vi "Main interface manual control.vi"(1 "Current":T1={"Pump 1 control"={"Pump Direction"=0, "Flow rate (ml/min)"=1.0, "Target volum (ml)"=1.0, "Run"=FALSE}, "Pump 4 control"={"Pump Direction"=0, "Flow rate (ml/min)"=1.0, "Target volum (ml)"=1.0, "Run"=FALSE}, "Pump 2 control"={"Flowrate (ml/min)"=0.0, "Target volume (ml)"=0.0, "Run"=FALSE}, "Pump 5 control"={"Pump Direction"=0, "Flow rate (ml/min)"=1.0, "Target volum (ml)"=1.0, "Run"=FALSE}, "Pump 3 control"={"Flowrate (ml/min)"=0.0, "Target volume (ml)"=0.0, "Run"=FALSE}} {"Pump 3 control"."Target volume (ml)" min=0.0 max=50.0 format="%#.3g"; "Pump 3 control"."Flowrate (ml/min)" min=0.0 max=500.0 format="%#.3g"; "Pump 5 control"."Target volum (ml)" format="%#.4f"; "Pump 5 control"."Flow rate (ml/min)" format="%#.4f"; "Pump 5 control"."Pump Direction" items=["Infuse", "Withdraw"]; "Pump 2 control"."Target volume (ml)" min=0.0 max=50.0 format="%#.3g"; "Pump 2 control"."Flowrate (ml/min)" min=0.0 max=500.0 format="%#.3g"; "Pump 4 control"."Target volum (ml)" format="%#.4f"; "Pump 4 control"."Flow rate (ml/min)" format="%#.4f"; "Pump 4 control"."Pump Direction" items=["Infuse", "Withdraw"]; "Pump 1 control"."Target volum (ml)" format="%#.4f"; "Pump 1 control"."Flow rate (ml/min)" format="%#.4f"; "Pump 1 control"."Pump Direction" items=["Infuse", "Withdraw"]}, 5 "Enable potentiostat":bool, 9 "Previous":T1={"Pump 1 control"={"Pump Direction"=0, "Flow rate (ml/min)"=1.0, "Target volum (ml)"=1.0, "Run"=FALSE}, "Pump 4 control"={"Pump Direction"=0, "Flow rate (ml/min)"=1.0, "Target volum (ml)"=1.0, "Run"=FALSE}, "Pump 2 control"={"Flowrate (ml/min)"=0.0, "Target volume (ml)"=0.0, "Run"=FALSE}, "Pump 5 control"={"Pump Direction"=0, "Flow rate (ml/min)"=1.0, "Target volum (ml)"=1.0, "Run"=FALSE}, "Pump 3 control"={"Flowrate (ml/min)"=0.0, "Target volume (ml)"=0.0, "Run"=FALSE}} {"Pump 3 control"."Target volume (ml)" min=0.0 max=50.0 format="%#.3g"; "Pump 3 control"."Flowrate (ml/min)" min=0.0 max=500.0 format="%#.3g"; "Pump 5 control"."Target volum (ml)" format="%#.4f"; "Pump 5 control"."Flow rate (ml/min)" format="%#.4f"; "Pump 5 control"."Pump Direction" items=["Infuse", "Withdraw"]; "Pump 2 control"."Target volume (ml)" min=0.0 max=50.0 format="%#.3g"; "Pump 2 control"."Flowrate (ml/min)" min=0.0 max=500.0 format="%#.3g"; "Pump 4 control"."Target volum (ml)" format="%#.4f"; "Pump 4 control"."Flow rate (ml/min)" format="%#.4f"; "Pump 4 control"."Pump Direction" items=["Infuse", "Withdraw"]; "Pump 1 control"."Target volum (ml)" format="%#.4f"; "Pump 1 control"."Flow rate (ml/min)" format="%#.4f"; "Pump 1 control"."Pump Direction" items=["Infuse", "Withdraw"]}, 11 "Configured COM ports":T2={"Pump 1 COM"="COM12", "Pump 2 COM"="COM9", "Pump 3 COM"="COM13", "Pump 4 COM"="COM4", "Pump 5 COM"="COM4"}) -> ()   [LabVIEW 2017]
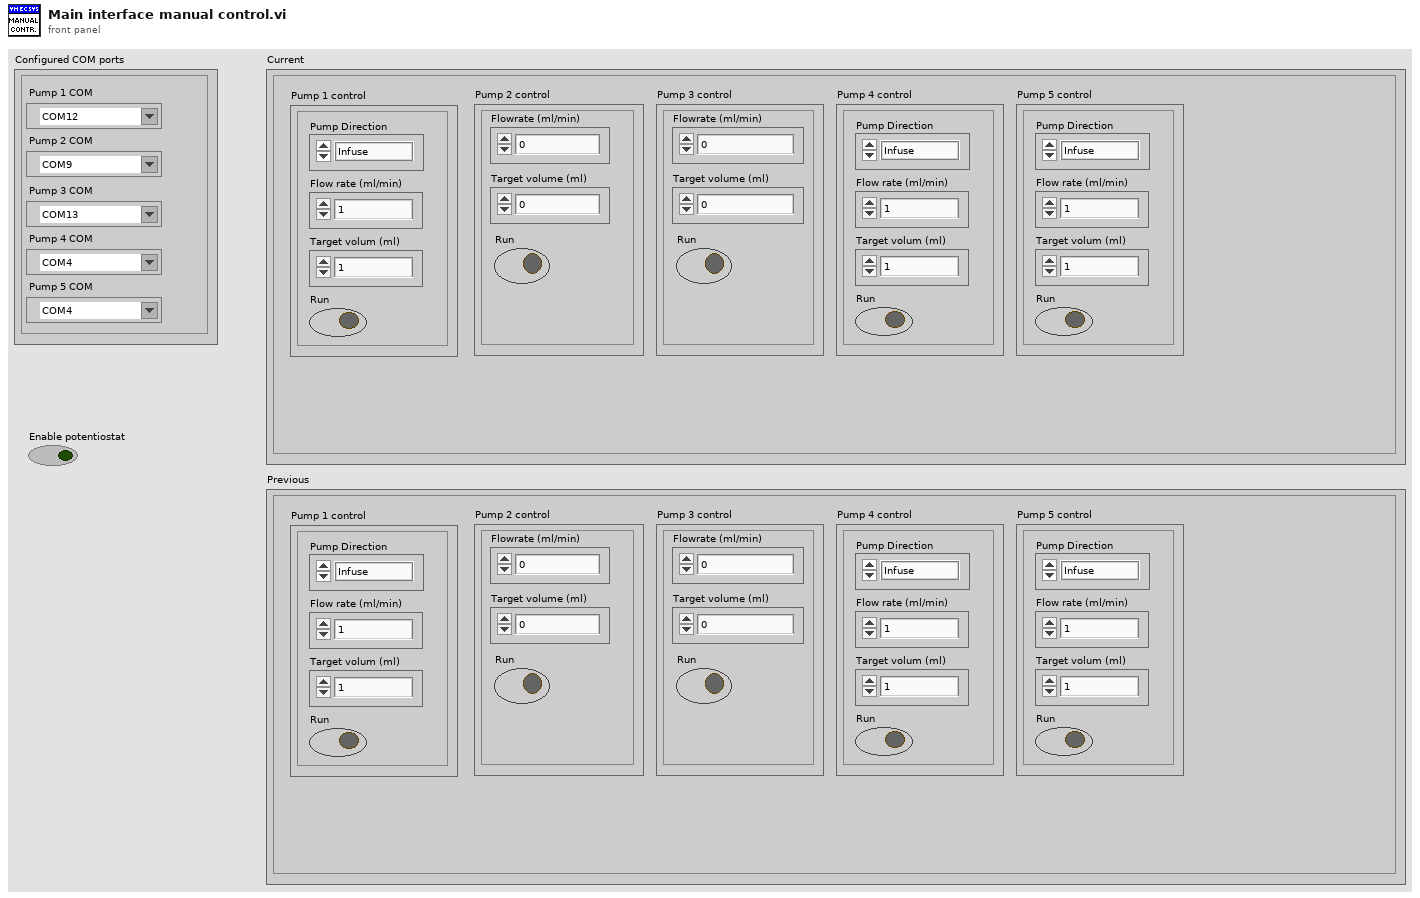
[diagram p1: front panel]
types:
  T1 = cluster{"Pump 1 control":cluster{"Pump Direction":u16, "Flow rate (ml/min)":dbl, "Target volum (ml)":dbl, "Run":bool}, "Pump 4 control":cluster{"Pump Direction":u16, "Flow rate (ml/min)":dbl, "Target volum (ml)":dbl, "Run":bool}, "Pump 2 control":cluster{"Flowrate (ml/min)":dbl, "Target volume (ml)":dbl, "Run":bool}, "Pump 5 control":cluster{"Pump Direction":u16, "Flow rate (ml/min)":dbl, "Target volum (ml)":dbl, "Run":bool}, "Pump 3 control":cluster{"Flowrate (ml/min)":dbl, "Target volume (ml)":dbl, "Run":bool}}
  T2 = cluster{"Pump 1 COM":refnum<visa-resource-name>, "Pump 2 COM":refnum<visa-resource-name>, "Pump 3 COM":refnum<visa-resource-name>, "Pump 4 COM":refnum<visa-resource-name>, "Pump 5 COM":refnum<visa-resource-name>}
  T3 = cluster{"Pump Direction":u16, "Flow rate (ml/min)":dbl, "Target volum (ml)":dbl, "Run":bool}
  T4 = cluster{"Flowrate (ml/min)":dbl, "Target volume (ml)":dbl, "Run":bool}
  T5 = cluster{"Pump Direction":bool, "Flow rate (ml/min)":bool, "Target volum (ml)":bool, "Run":bool}
  T6 = cluster{"Flowrate (ml/min)":bool, "Target volume (ml)":bool, "Run":bool}
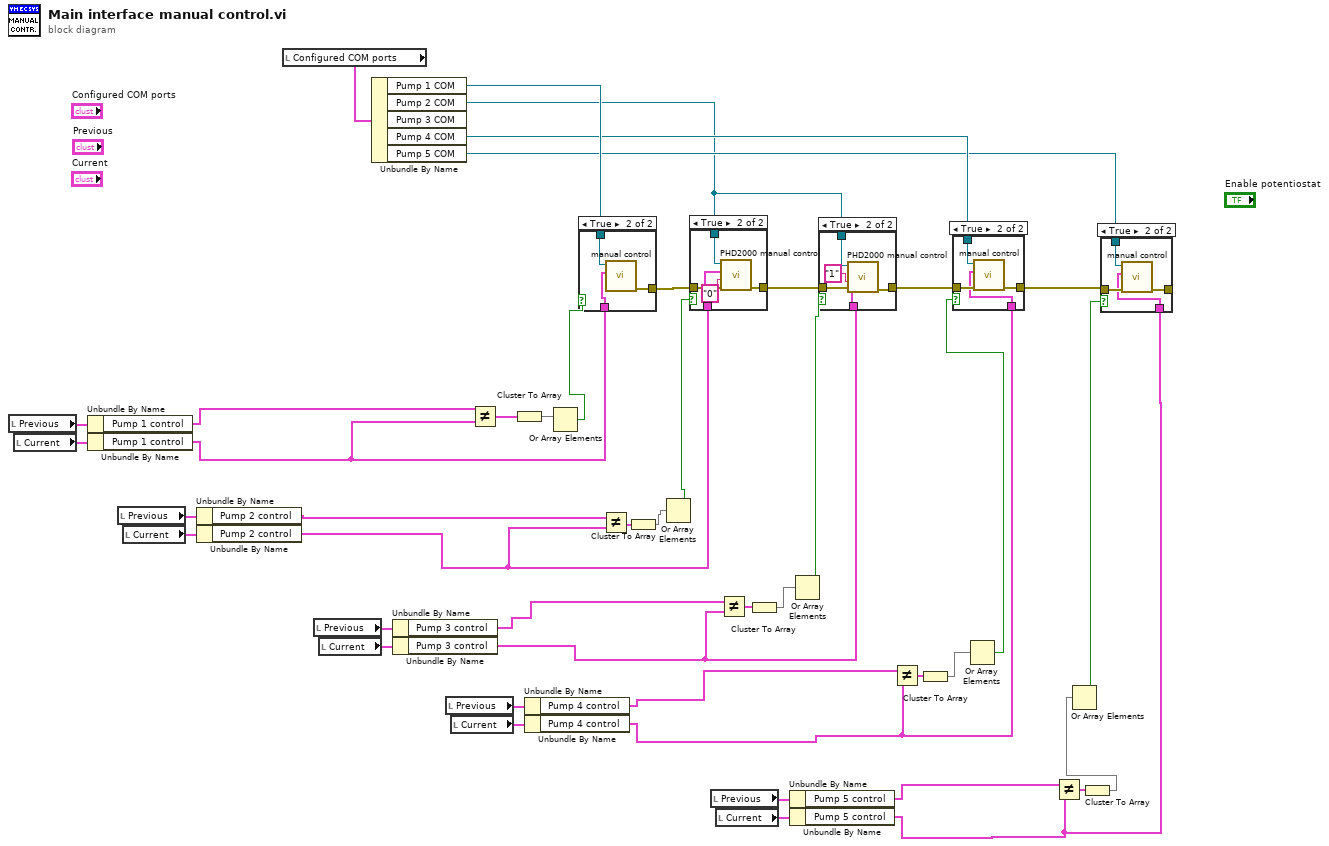
[diagram p0: block diagram]
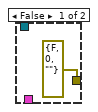
[diagram p6: hidden frame]
diagram:
  n1 = local read "Previous"() -> (w18:T1)
  n2 = local read "Current"() -> (w17:T1)
  n3 = Unbundle By Name(w18) -> ("Pump 1 control"=w20:T3)
  n4 = Unbundle By Name(w17) -> ("Pump 1 control"=w19:T3)
  n5 = local read "Previous"() -> (w15:T1)
  n6 = local read "Current"() -> (w16:T1)
  n7 = Unbundle By Name(w15) -> ("Pump 2 control"=w1:T4)
  n8 = Unbundle By Name(w16) -> ("Pump 2 control"=w2:T4)
  n9 = local read "Configured COM ports"() -> (w44:T2)
  n10 = local read "Previous"() -> (w14:T1)
  n11 = local read "Current"() -> (w13:T1)
  n12 = Unbundle By Name(w44) -> ("Pump 1 COM"=w43:refnum<visa-resource-name>, "Pump 2 COM"=w23:refnum<visa-resource-name>, "Pump 4 COM"=w42:refnum<visa-resource-name>, "Pump 5 COM"=w25:refnum<visa-resource-name>)  [unwired: 1 out]
  n13 = Unbundle By Name(w14) -> ("Pump 3 control"=w3:T4)
  n14 = Unbundle By Name(w13) -> ("Pump 3 control"=w4:T4)
  n15 = local read "Previous"() -> (w11:T1)
  n16 = local read "Current"() -> (w12:T1)
  n17 = Not Equal?(x=w20, y=w19) -> (x != y?=w38:T5)
  n18 = Cluster To Array(cluster=w38) -> (array=w35:bool[])
  n19 = Unbundle By Name(w11) -> ("Pump 4 control"=w5:T3)
  n20 = Unbundle By Name(w12) -> ("Pump 4 control"=w6:T3)
  n21 = Or Array Elements(Boolean array=w35) -> (logical OR=w34:bool)
  n22 = case shown="True" w34 {
    tunnel: w43 -> [_ w48]
    tunnel: [errorcluster {"status"=FALSE, "code"=0, "source"=""} ("error out") w47] -> w41
    tunnel: w19 -> [_ w46]
    frame False {
    }
    frame True {
      n23 = call "manual control.vi"("control"=w46, "VISA resource name"=w48) -> ("error out"=w47:errorcluster)  [unwired: 8 in, 1 out]
    }
  }
  n24 = Not Equal?(x=w1, y=w2) -> (x != y?=w37:T6)
  n25 = Cluster To Array(cluster=w37) -> (array=w33:bool[])
  n26 = Or Array Elements(Boolean array=w33) -> (logical OR=w30:bool)
  n27 = case shown="True" w30 {
    tunnel: w41 -> [w49 w54]
    tunnel: [w49 w53] -> w40
    tunnel: w23 -> [_ w52]
    tunnel: w2 -> [_ w51]
    frame False {
    }
    frame True {
      n28 = call "PHD2000 manual control.vi"("error in (no error)"=w54, "Pump #"="0", "control"=w51, "VISA resource name 2"=w52) -> ("error out"=w53:errorcluster)  [unwired: 6 in, 1 out]
    }
  }
  n29 = local read "Previous"() -> (w10:T1)
  n30 = local read "Current"() -> (w9:T1)
  n31 = Not Equal?(x=w3, y=w4) -> (x != y?=w21:T6)
  n32 = Cluster To Array(cluster=w21) -> (array=w22:bool[])
  n33 = Unbundle By Name(w10) -> ("Pump 5 control"=w8:T3)
  n34 = Unbundle By Name(w9) -> ("Pump 5 control"=w7:T3)
  n35 = Or Array Elements(Boolean array=w22) -> (logical OR=w31:bool)
  n36 = case shown="True" w31 {
    tunnel: w40 -> [w55 w58]
    tunnel: [w55 w59] -> w39
    tunnel: w23 -> [_ w60]
    tunnel: w4 -> [_ w56]
    frame False {
    }
    frame True {
      n37 = call "PHD2000 manual control.vi"("error in (no error)"=w58, "Pump #"="1", "control"=w56, "VISA resource name 2"=w60) -> ("error out"=w59:errorcluster)  [unwired: 6 in, 1 out]
    }
  }
  n38 = Not Equal?(x=w5, y=w6) -> (x != y?=w36:T5)
  n39 = Cluster To Array(cluster=w36) -> (array=w32:bool[])
  n40 = Or Array Elements(Boolean array=w32) -> (logical OR=w29:bool)
  n41 = case shown="True" w29 {
    tunnel: w42 -> [_ w65]
    tunnel: w39 -> [w61 w64]
    tunnel: w6 -> [_ w63]
    tunnel: [w61 w62] -> w24
    frame False {
    }
    frame True {
      n42 = call "manual control.vi"("error in (no error)"=w64, "control"=w63, "VISA resource name"=w65) -> ("error out"=w62:errorcluster)  [unwired: 7 in, 1 out]
    }
  }
  n43 = Not Equal?(x=w8, y=w7) -> (x != y?=w28:T5)
  n44 = Cluster To Array(cluster=w28) -> (array=w27:bool[])
  n45 = Or Array Elements(Boolean array=w27) -> (logical OR=w26:bool)
  n46 = case shown="True" w26 {
    tunnel: w25 -> [_ w70]
    tunnel: w24 -> [w66 w69]
    tunnel: w7 -> [_ w68]
    tunnel: [w66 w67] -> _
    frame False {
    }
    frame True {
      n47 = call "manual control.vi"("error in (no error)"=w69, "control"=w68, "VISA resource name"=w70) -> ("error out"=w67:errorcluster)  [unwired: 7 in, 1 out]
    }
  }
